vi "Obtain Messaging Network.vi"(8 "error in (no error)":errorcluster) -> (0 "error out":errorcluster, 3 "msg cluster":T1)   [LabVIEW 2020]
uses:
  Messaging Cluster.ctl
  Hardware/Sensors/Cameras/Camera.lvclass
  Hardware/Sensors/Force Sensors/Force Sensor.lvclass
  Hardware/Actuators/Servos/Servo.lvclass
  Hardware/Actuators/Switches/Switch.lvclass
  Controller Loop/Message and Data.ctl
  Inflation Test/Parameter Class/IA Test Parameters.lvclass
  Controllers/Controller.lvclass
  File Interfacing/Filename Structure.ctl
  GUI/Main GUI Loop/Handler.ctl
  Inflation Test/Result Handling/Inflation Test Numeric Results.ctl
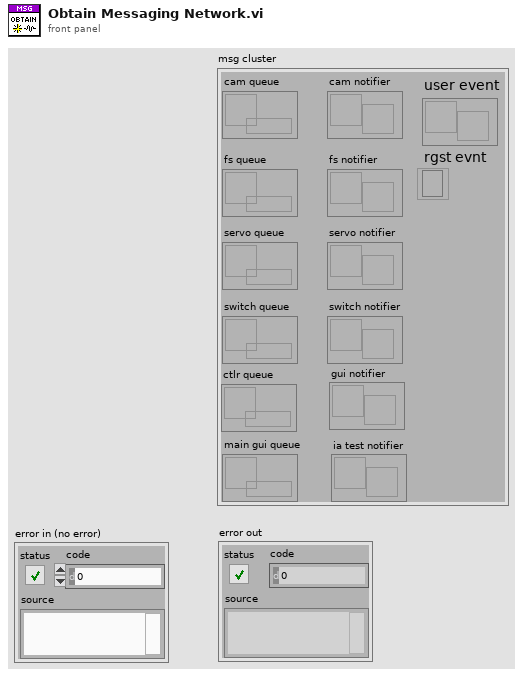
[diagram p1: front panel]
types:
  T1 = typedef "Messaging Cluster.ctl" = cluster{"cam queue":refnum<queue>, "fs queue":refnum<queue>, "servo queue":refnum<queue>, "switch queue":refnum<queue>, "switch notifier":refnum<notifier>, "servo notifier":refnum<notifier>, "fs notifier":refnum<notifier>, "cam notifier":refnum<notifier>, "rgst evnt":refnum<event-registration>, "user event":refnum<user-event>, "ctlr queue":refnum<queue>, "main gui queue":refnum<queue>, "gui notifier":refnum<notifier>, "ia test notifier":refnum<notifier>}
  T2 = typedef "Inflation Test Numeric Results.ctl" = cluster{"diameter":dbl, "diam time":dbl, "force":dbl, "force time":dbl, "setpoint":dbl, "servo pw":dbl, "calibration log":dbl[][], "calibration results":dbl[][]}
  T3 = typedef "Handler.ctl" = cluster{"bool ref":refnum<vi>, "error":errorcluster, "msg":string, "status":string, "switch status":bool, "force cal":dbl[][], "force cal results":dbl[][]}
  T4 = typedef "Message and Data.ctl" = cluster{"msg":string, "ia test param":refnum<class "IA Test Parameters.lvclass">, "controller type":refnum<class "Controller.lvclass">, "folder path":path, "file name":string, "file comments":string, "cam":refnum<class "Camera.lvclass">, "fs":refnum<class "Force Sensor.lvclass">, "servo":refnum<class "Servo.lvclass">, "switch":refnum<class "Switch.lvclass">, "filename struct":T5}
  T5 = typedef "Filename Structure.ctl" = enum16{"<nameYYYYMMDDi>", "<name>"}
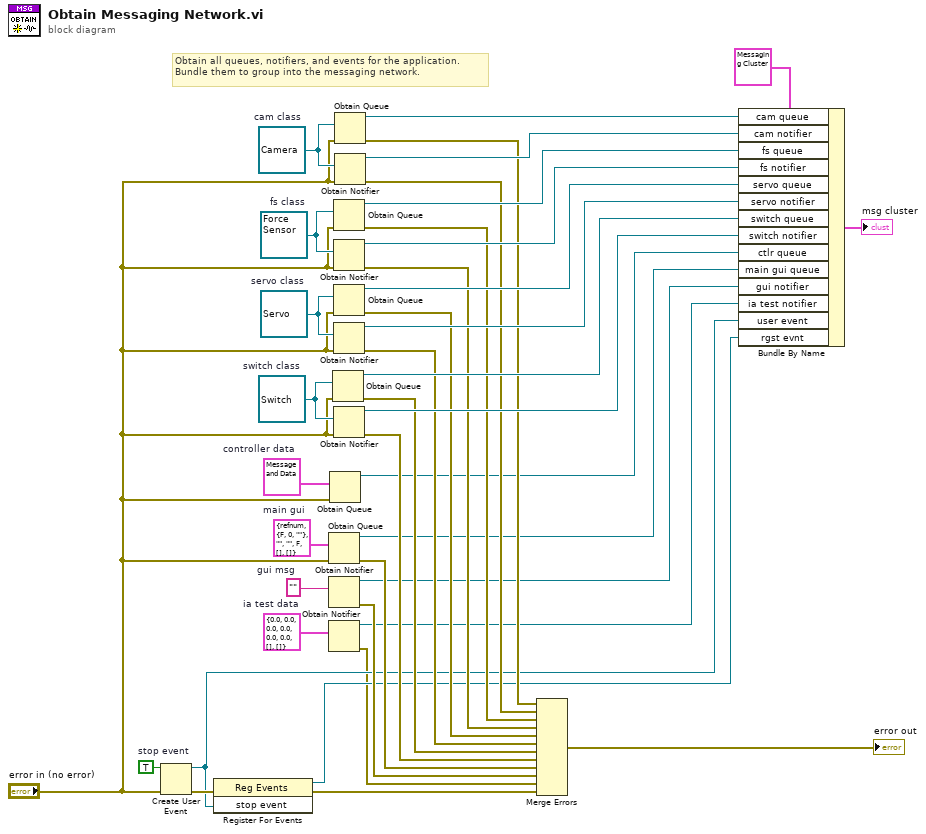
[diagram p0: block diagram]
diagram:
  w4 = T2 {"diameter"=0.0, "diam time"=0.0, "force"=0.0, "force time"=0.0, "setpoint"=0.0, "servo pw"=0.0, "calibration log"=[], "calibration results"=[]}  # ia test data
  w8 = ""  # gui msg
  w12 = T3 {"bool ref"=refnum, "error"={"status"=FALSE, "code"=0, "source"=""}, "msg"="", "status"="", "switch status"=FALSE, "force cal"=[], "force cal results"=[]}  # main gui
  w15 = T4 {"msg"="", "ia test param"=refnum, "controller type"=refnum, "folder path"=path "", "file name"="", "file comments"="", "cam"=refnum, "fs"=refnum, "servo"=refnum, "switch"=refnum, "filename struct"=enum."<nameYYYYMMDDi>"}  # controller data
  w16 = TRUE  # stop event
  w33 = refnum<class "Force Sensor.lvclass"> refnum  # fs class
  w34 = refnum<class "Camera.lvclass"> refnum  # cam class
  w35 = refnum<class "Servo.lvclass"> refnum  # servo class
  w36 = refnum<class "Switch.lvclass"> refnum  # switch class
  # "Obtain all queues, notifiers, and events for the application. Bundle them to group into the messaging network."
  n1 = Create User Event(user event datatype=w16, error in="error in (no error)") -> (user event=w5:refnum<user-event>, error out=w17:errorcluster)
  n2 = register-events(error in=w17, w5) -> (reference out=w6:refnum<event-registration>, error out=w2:errorcluster)  [unwired: 1 in]
  n3 = Obtain Queue(element data type=w12, error in (no error)="error in (no error)") -> (queue out=w11:refnum<queue>, error out=w13:errorcluster)  [unwired: 3 in, 1 out]
  n4 = Obtain Notifier(notification data type=w8) -> (notifier out=w7:refnum<notifier>, error out=w9:errorcluster)  [unwired: 3 in, 1 out]
  n5 = Obtain Notifier(notification data type=w4) -> (notifier out=w3:refnum<notifier>, error out=w1:errorcluster)  [unwired: 3 in, 1 out]
  n6 = Obtain Queue(element data type=w15, error in (no error)="error in (no error)") -> (queue out=w14:refnum<queue>)  [unwired: 3 in, 2 out]
  n7 = Obtain Queue(element data type=w36, error in (no error)="error in (no error)") -> (queue out=w27:refnum<queue>, error out=w24:errorcluster)  [unwired: 3 in, 1 out]
  n8 = Obtain Queue(element data type=w33, error in (no error)="error in (no error)") -> (queue out=w31:refnum<queue>, error out=w20:errorcluster)  [unwired: 3 in, 1 out]
  n9 = Obtain Notifier(notification data type=w33, error in (no error)="error in (no error)") -> (notifier out=w30:refnum<notifier>, error out=w21:errorcluster)  [unwired: 2 in, 1 out]
  n10 = Obtain Queue(element data type=w35, error in (no error)="error in (no error)") -> (queue out=w29:refnum<queue>, error out=w22:errorcluster)  [unwired: 3 in, 1 out]
  n11 = Obtain Notifier(notification data type=w35, error in (no error)="error in (no error)") -> (notifier out=w28:refnum<notifier>, error out=w23:errorcluster)  [unwired: 2 in, 1 out]
  n12 = Obtain Notifier(notification data type=w36, error in (no error)="error in (no error)") -> (notifier out=w26:refnum<notifier>, error out=w25:errorcluster)  [unwired: 2 in, 1 out]
  n13 = Obtain Queue(element data type=w34, error in (no error)="error in (no error)") -> (queue out=w39:refnum<queue>, error out=w18:errorcluster)  [unwired: 3 in, 1 out]
  n14 = Obtain Notifier(notification data type=w34, error in (no error)="error in (no error)") -> (notifier out=w32:refnum<notifier>, error out=w19:errorcluster)  [unwired: 2 in, 1 out]
  n15 = Merge Errors(w18, w19, w20, w21, w22, w23, w24, w25, w13, w9, w1, w2) -> (→"error out":errorcluster)
  n16 = Bundle By Name(cluster=T1 {"cam queue"=refnum, "fs queue"=refnum, "servo queue"=refnum, "switch queue"=refnum, "switch notifier"=refnum, "servo notifier"=refnum, "fs notifier"=refnum, "cam notifier"=refnum, "rgst evnt"=refnum, "user event"=refnum, "ctlr queue"=refnum, "main gui queue"=refnum, "gui notifier"=refnum, "ia test notifier"=refnum}, "cam queue"=w39, "cam notifier"=w32, "fs queue"=w31, "fs notifier"=w30, "servo queue"=w29, "servo notifier"=w28, "switch queue"=w27, "switch notifier"=w26, "ctlr queue"=w14, "main gui queue"=w11, "gui notifier"=w7, "ia test notifier"=w3, "user event"=w5, "rgst evnt"=w6) -> (→"msg cluster":T1)
